vi "Recursive Search and Replace.vi"(7 "Replacement Channels":T1={"Channel to Replace"="Targets/Controller/Custom Devices/VCOM/CAN_Sender_Tx/ACC/ACC_ESP_E2E_PR2/ACC_NEW_SIGNAL", "Replacement Channel"="Targets/Controller/User Channels/User Channel 1"}, 8 "error in (no error)":errorcluster, 9 "Data Source Nodes In":string[](array[string]), 11 ".NET Refnum":refnum<k24>) -> (0 "error out":errorcluster, 2 "Replacement Log":string[](array[string]))   [LabVIEW 2025]
uses:
  Replacement Channels.ctl
  NationalInstruments.VeriStand.SystemDefinitionAPI
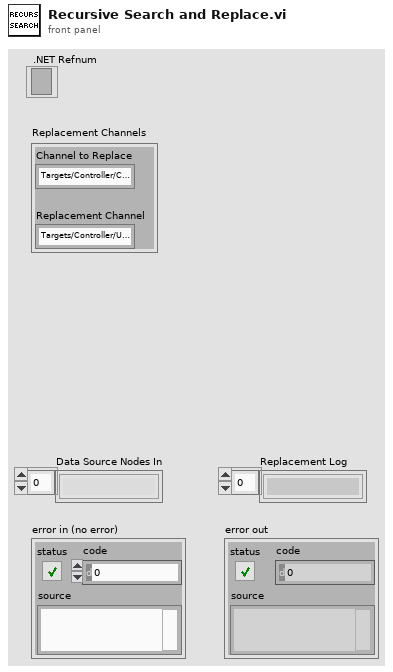
[diagram p1: front panel]
types:
  T1 = typedef "Replacement Channels.ctl" = cluster{"Channel to Replace":string, "Replacement Channel":string}
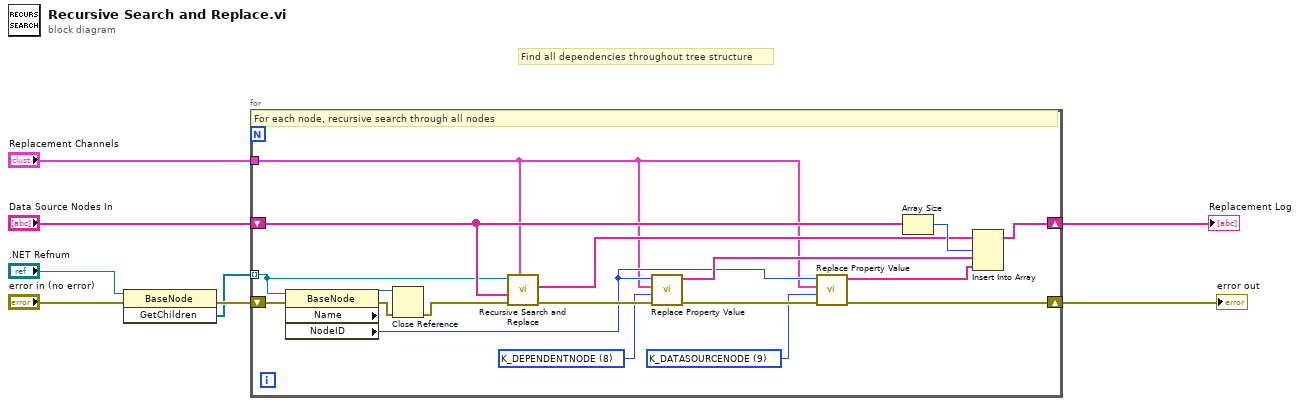
[diagram p0: block diagram]
diagram:
  # "Find all dependencies throughout tree structure"
  n1 = invoke class="BaseNode" method="GetChildren"(reference=".NET Refnum", error in="error in (no error)") -> (error out=w7:errorcluster, "GetChildren"=w1:refnum<k24>[])  [unwired: 1 in, 1 out]
  n2 = for {
    shift-right: [w14] -> w5
    shift-left: w7 -> [w26]
    shift-right: [w24] -> w4
    shift-left: "Data Source Nodes In" -> [w23]
    tunnel: "Replacement Channels" -> [w15]
    tunnel: w1 -> [w12] mode=indexing
    w17 = 9 items=["K_STRING", "K_BOOL", "K_I32", "K_U32", "K_DOUBLE", "K_U64", "K_VARIANT", "K_DEPENDENTFILE", "K_DEPENDENTNODE", "K_DATASOURCENODE", "K_U16", "K_DBLARR", "K_U32ARR", "K_I32ARR", "K_STRINGARR", "K_DICTIONARY", "K_DICTIONARYARR", "K_BINARYSTRING", "K_I16", "K_I64", "K_BOOLARR", "K_U64ARR", "K_U16ARR", "K_I64ARR", "K_I16ARR"] ("Property Type")
    w19 = 8 items=["K_STRING", "K_BOOL", "K_I32", "K_U32", "K_DOUBLE", "K_U64", "K_VARIANT", "K_DEPENDENTFILE", "K_DEPENDENTNODE", "K_DATASOURCENODE", "K_U16", "K_DBLARR", "K_U32ARR", "K_I32ARR", "K_STRINGARR", "K_DICTIONARY", "K_DICTIONARYARR", "K_BINARYSTRING", "K_I16", "K_I64", "K_BOOLARR", "K_U64ARR", "K_U16ARR", "K_I64ARR", "K_I16ARR"] ("Property Type")
    # "For each node, recursive search through all nodes"
    n3 = property class="BaseNode" props=["Name", "NodeID"](reference=w12, error in=w26) -> (reference out=w10:refnum<k24>, error out=w11:errorcluster, "NodeID"=w16:u64)  [unwired: 1 out]
    n4 = Close Reference(reference=w10, error in (no error)=w11) -> (error out=w9:errorcluster)
    n5 = call "Recursive Search and Replace.vi"("Replacement Channels"=w15, "error in (no error)"=w9, "Data Source Nodes In"=w23, ".NET Refnum"=w12) -> ("error out"=w20:errorcluster, "Replacement Log"=w22:string[])  [unwired: 6 in]
    n6 = call "Replace Property Value.vi"("error in (no error)"=w20, "Property Type"=w19, "Replacement Channels"=w15, "NodeID"=w16) -> ("error out"=w18:errorcluster, "Replacement Log"=w21:string[])  [unwired: 6 in]
    n7 = call "Replace Property Value.vi"("error in (no error)"=w18, "Property Type"=w17, "Replacement Channels"=w15, "NodeID"=w16) -> ("error out"=w14:errorcluster, "Replacement Log"=w13:string[])  [unwired: 6 in]
    n8 = Array Size(array=w23) -> (size(s)=w25:i32)
    n9 = Insert Into Array(array=w22, index=w25, new element #1=w21, new element #2=w13) -> (w24:string[])
  }
  "error out" <- w5
  "Replacement Log" <- w4
